vi "Mouse Breathing Monitor V6.vi"() -> ()   [LabVIEW 2017]
uses:
  <vilib>/Utility/error.llb/DialogType.ctl
  <vilib>/Utility/sysdir.llb/System Directory Type.ctl
  C:/Program Files (x86)/National Instruments/LabVIEW 2017/vi.lib/ULx/ULx_LV.dll
  Program Files (x86)/National Instruments/LabVIEW 2017/vi.lib/ULx/ULx_LV.dll
  <vilib>/Analysis/baseanly.llb/Mean (DBL).vi
  <vilib>/ULx/Create Channel.llb/ULx Create Channel (AI-Voltage-Basic).vi
  <vilib>/ULx/Timing.llb/ULx Timing (Sample Clock).vi
  <vilib>/ULx/Read.llb/ULx Read (Analog 2D DBL NChan NSamp).vi
  <vilib>/Analysis/NI_AALBase.lvlib
panel:
  in  "CH 2 Calibration Volume (mL)":dbl min=0.0 max=0.5 format="%#_13g"
  in  "CH 1 Calibration Volume (mL)":dbl min=0.0 max=0.5 format="%#_13g"
  in  "CH2 Cuff Alarm Threshold":dbl=3.0
  out "CH2 Cuff Alarm":bool
  in  "CH1 Cuff Alarm Threshold":dbl=3.0
  out "CH1 Cuff Alarm":bool
  out "CH1 Cuff":dbl format="%0.2f"
  out "CH2 Cuff":dbl format="%0.2f"
  in  "Invert Signal?":bool=TRUE
  in  "CH2 Log Button":bool
  in  "CH2 Logging":bool
  in  "CH2 Record\nButton":bool
  in  "CH1 Record\nButton":bool
  in  "CH2 Mouse ID":string
  in  "CH2 Recording":bool
  in  "CH1 Recording":bool
  in  "CH2 refnum":refnum<file>
  in  "Seconds to Display":i32=5 min=1
  in  "CH1 Logging":bool
  in  "CH1 Log Button":bool
  in  "CH1 refnum":refnum<file>
  in  "Exit":bool
  in  "CH1 Mouse ID":string
  in  "Stop":bool
  out "CH2 Chart":dbl[](graph)=[4.998778820037842, 4.998778820037842, 4.998778820037842, 5.00122082256712, 4.998778820037842, 4.998778820037842, 4.998778820037842, 4.998778820037842, 4.998778820037842, 5.00122082256712]
  out "CH1 Chart":dbl[](graph)=[4.998778820037842, 5.00122082256712, 4.998778820037842, 4.998778820037842, 5.00122082256712, 4.998778820037842, 5.00122082256712, 4.998778820037842, 4.998778820037842, 5.00122082256712]
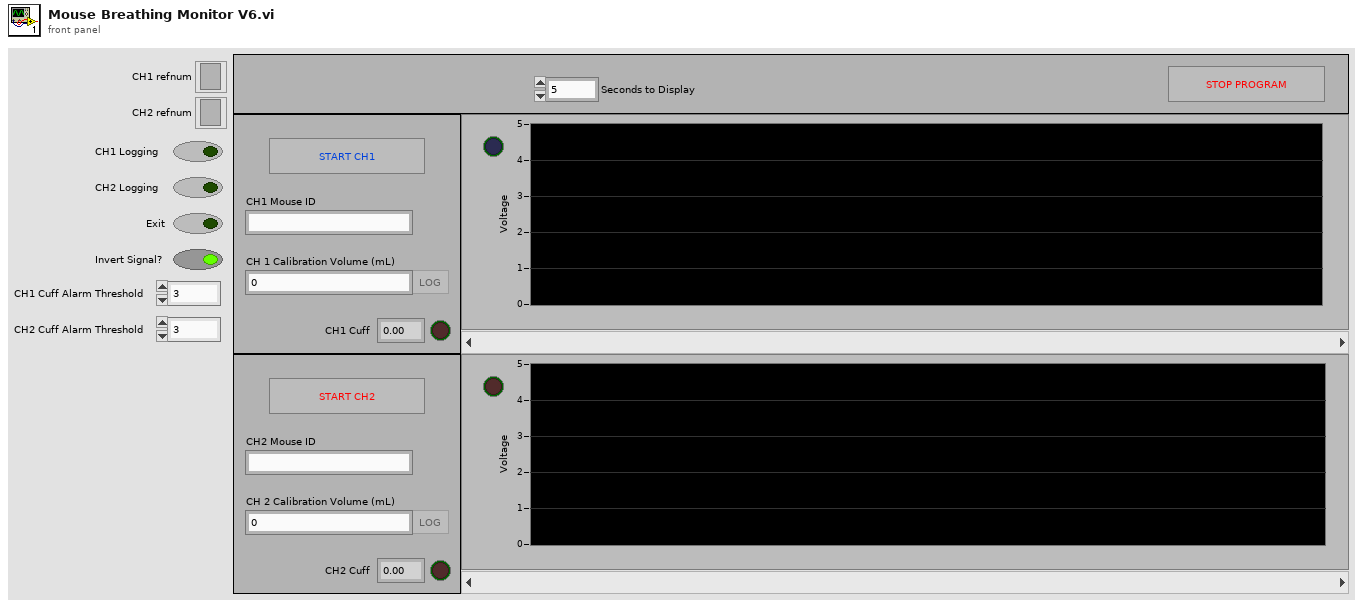
[diagram p1: front panel]
types:
  T1 = typedef "System Directory Type.ctl" = i32
  T2 = typedef "DialogType.ctl" = u16
  T3 = enum8{"Enabled", "Disabled", "Disabled and Grayed Out"}
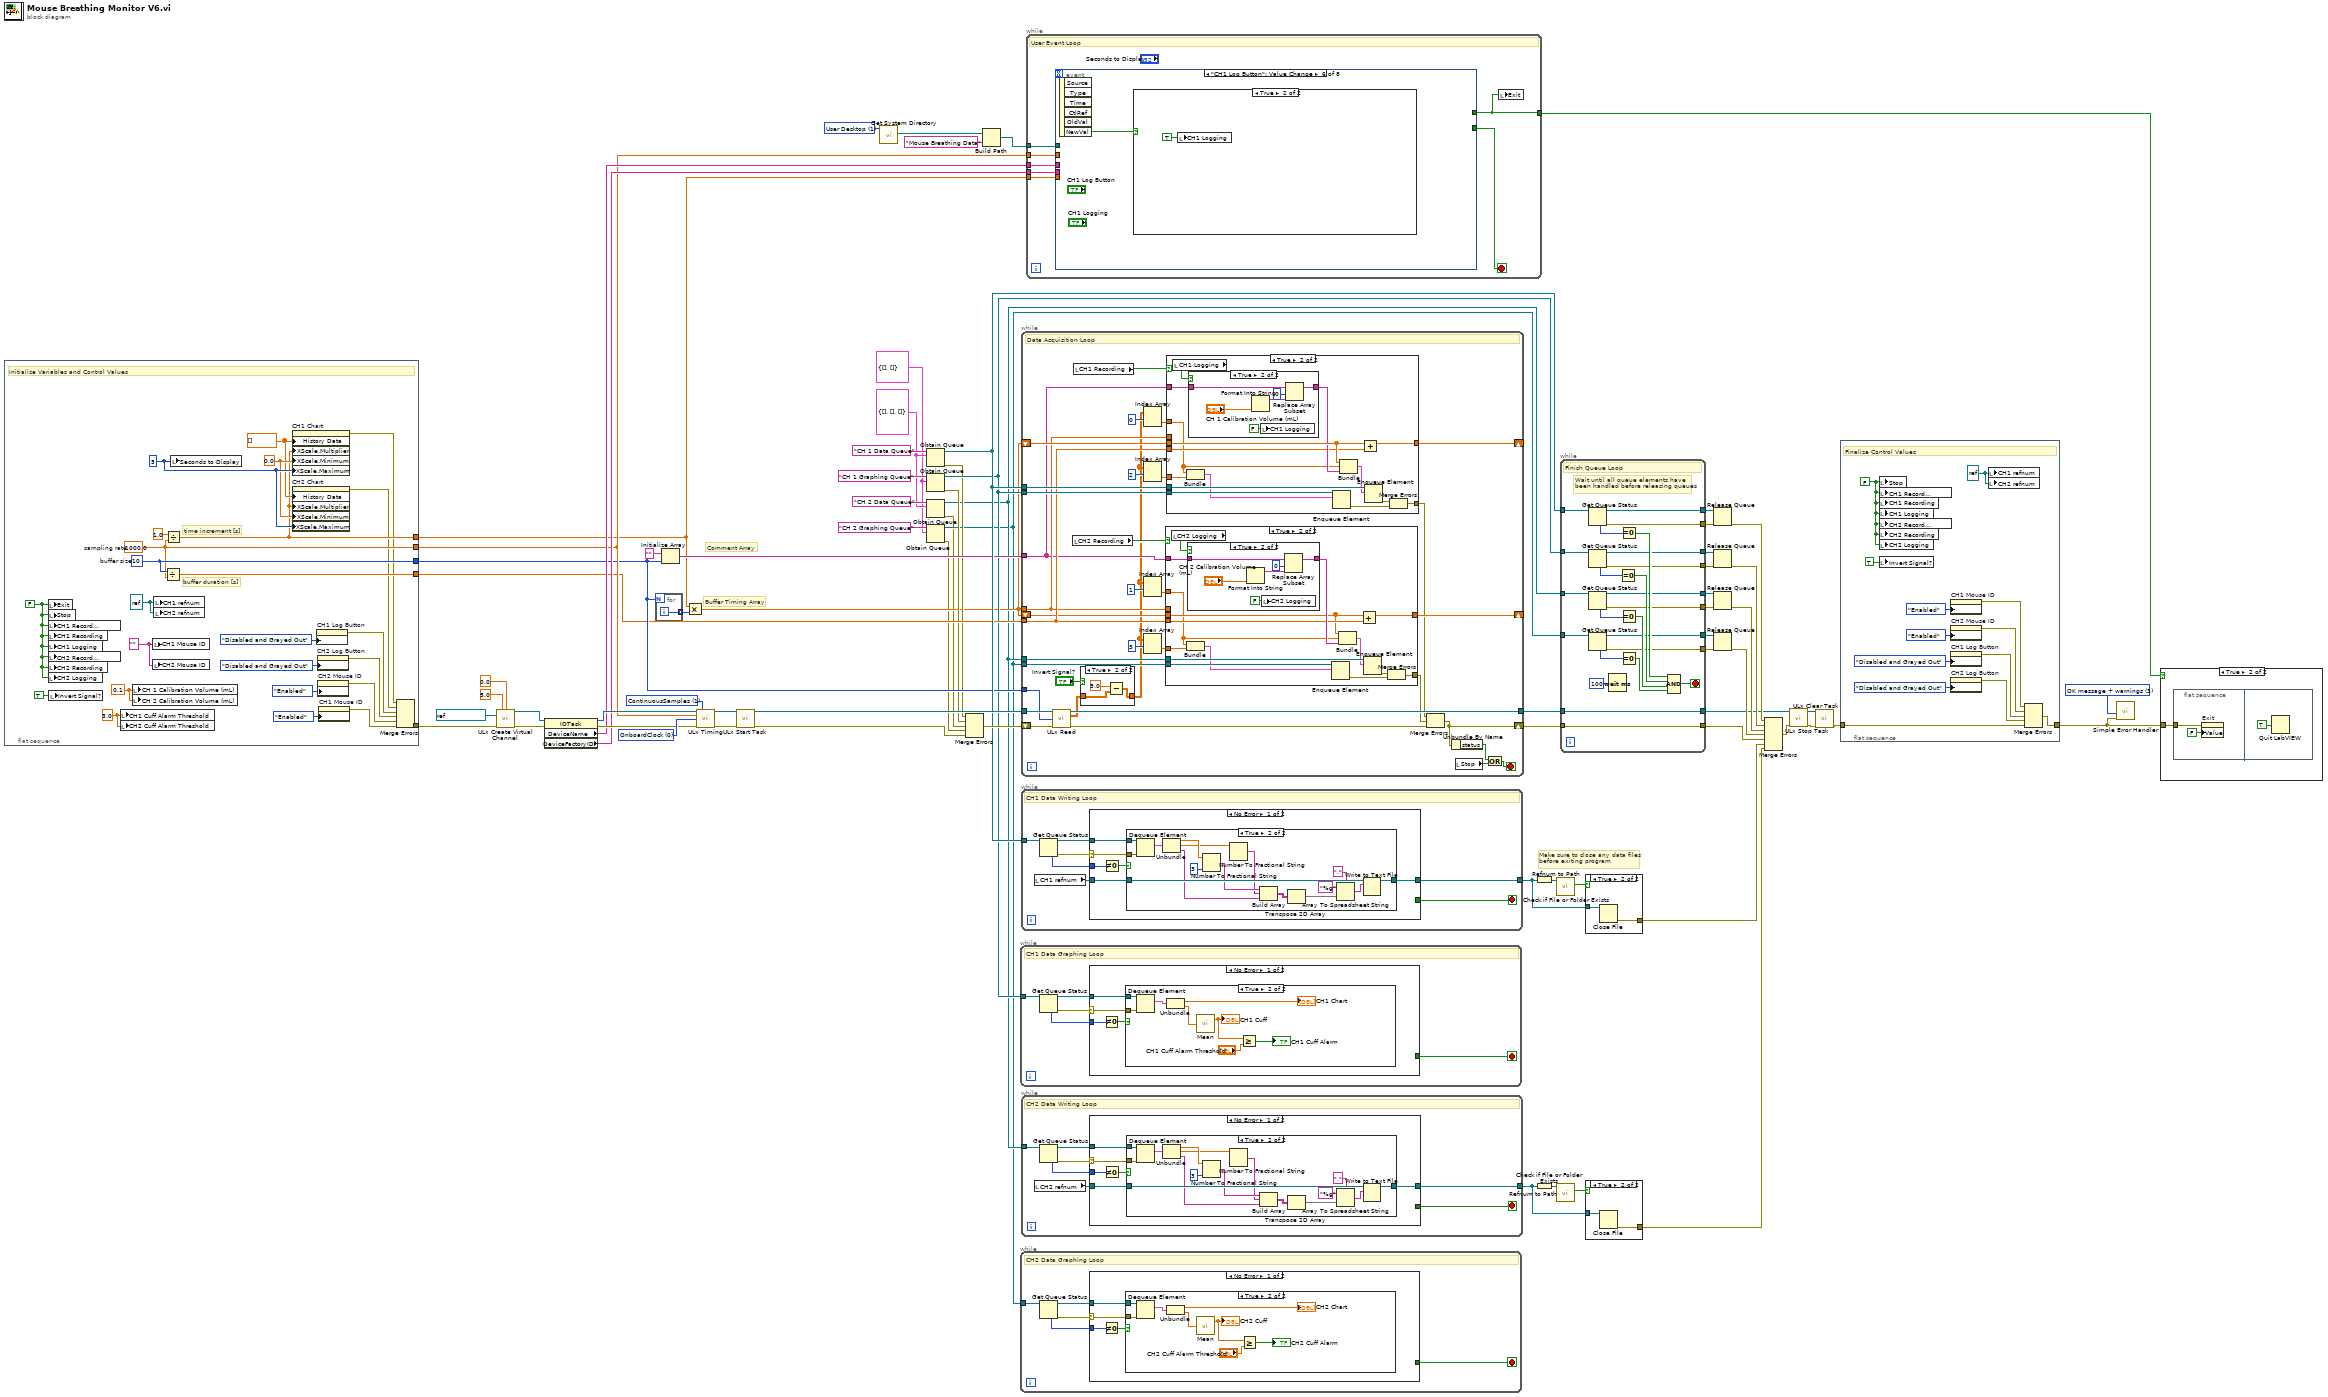
[diagram p0: block diagram]
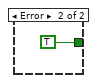
[diagram p4: hidden frame]
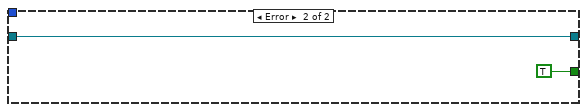
[diagram p6: hidden frame]
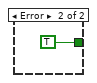
[diagram p8: hidden frame]
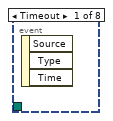
[diagram p11: hidden frame]
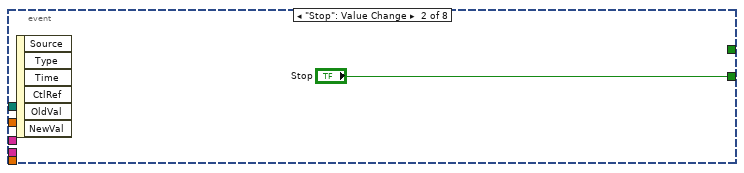
[diagram p12: hidden frame]
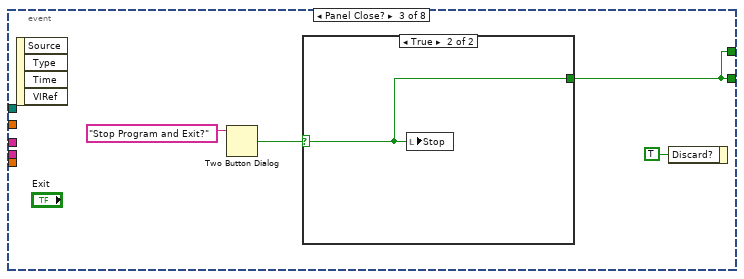
[diagram p13: hidden frame]
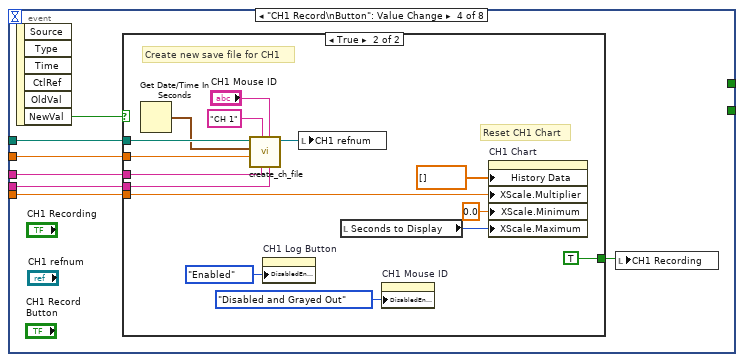
[diagram p15: hidden frame]
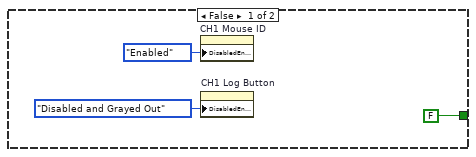
[diagram p16: hidden frame]
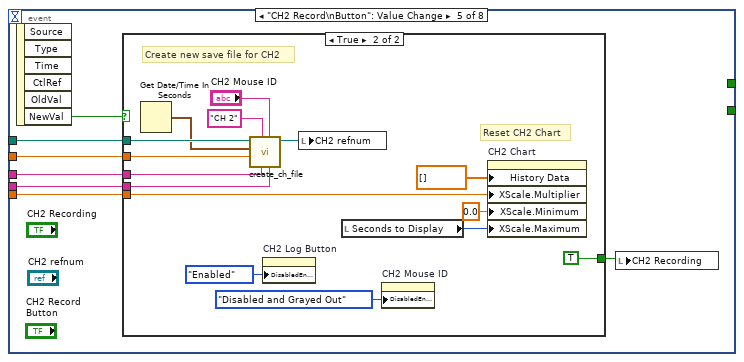
[diagram p17: hidden frame]
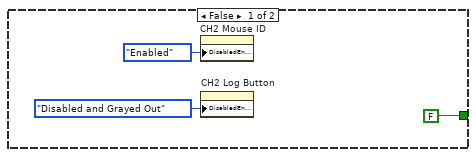
[diagram p18: hidden frame]
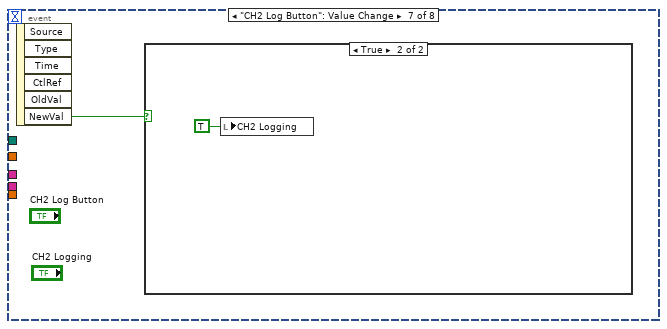
[diagram p20: hidden frame]
diagram:
  w1 = cluster{dbl[], dbl[]} {[], []}
  w32 = cluster{dbl[], dbl[], string[]} {[], [], []}
  w61 = T1 1 items=["User Home"=0, "User Desktop"=1, "User Documents"=2, "User Application Data"=3, "User Preferences"=4, "User Temporary"=5, "Public Documents"=6, "Public Application Data"=7, "Public Preferences"=8, "Public Cache"=13, "System Core Libraries"=9, "System Installed Libraries"=10, "Application Files"=11, "Boot Volume Root"=12] ("system directory type")
  w62 = 1 items=["FiniteSamples", "ContinuousSamples"] ("sample mode")
  w63 = 0 items=["OnboardClock", "ExternalClock", "NoClock"] ("clock source")
  w71 = T2 3 items=["no dialog", "OK message", "continue or stop message", "OK message + warnings", "continue/stop + warnings"] ("type of dialog (OK msg:1)")
  # "Make sure to close any data files\nbefore exiting program"
  # "Comment Array"
  # "Buffer Timing Array"
  n1 = flat-sequence {
    tunnel: [w89] -> w50
    tunnel: [w96] -> w45
    tunnel: [w97] -> w44
    tunnel: [w79] -> w43
    tunnel: [w95] -> w42
    frame #0 {
      w75 = 0.1 ("CH 1 Calibration Volume (mL)")
      w76 = 3.0
      w84 = refnum<file> refnum ("CH 1 refnum")
      w81 = 0.0 ("X Scale.Range:Minimum")
      w82 = 5 ("Seconds to Display")
      w80 = dbl[] [] ("CH1 Chart")
      w85 = "" ("CH 1 Mouse ID")
      w92 = FALSE ("Exit")
      w97 = 10  # buffer size
      w96 = 1000.0  # sampling rate
      # "buffer duration [s]"
      # "time increment [s]"
      # "Initialize Variables and Control Values"
      n2 = local write "Exit"(w92) -> ()
      n3 = local write "Stop"(w92) -> ()
      n4 = local write "CH1 Record\nButton"(w92) -> ()
      n5 = local write "CH1 Recording"(w92) -> ()
      n6 = local write "CH1 Logging"(w92) -> ()
      n7 = local write "CH2 Record\nButton"(w92) -> ()
      n8 = local write "CH2 Recording"(w92) -> ()
      n9 = local write "CH2 Logging"(w92) -> ()
      n10 = local write "Invert Signal?"(TRUE ("Invert Signal?")) -> ()
      n11 = local write "CH1 Cuff Alarm Threshold"(w76) -> ()
      n12 = local write "CH2 Cuff Alarm Threshold"(w76) -> ()
      n13 = local write "CH 1 Calibration Volume (mL)"(w75) -> ()
      n14 = local write "CH 2 Calibration Volume (mL)"(w75) -> ()
      n15 = local write "CH1 Mouse ID"(w85) -> ()
      n16 = local write "CH2 Mouse ID"(w85) -> ()
      n17 = local write "CH1 refnum"(w84) -> ()
      n18 = local write "CH2 refnum"(w84) -> ()
      n19 = Divide(x=w97, y=w96) -> (x/y=w95:dbl)
      n20 = Divide(x=1.0, y=w96) -> (x/y=w79:dbl)
      n21 = local write "Seconds to Display"(w82) -> ()
      n22 = property on="CH1 Chart" class="WFChart (strict)"("History Data"=w80, "XScale.Multiplier"=w79, "XScale.Minimum"=w81, "XScale.Maximum"=w82) -> (error out=w78:errorcluster)  [unwired: 2 in, 1 out]
      n23 = property on="CH2 Chart" class="WFChart (strict)"("History Data"=w80, "XScale.Multiplier"=w79, "XScale.Minimum"=w81, "XScale.Maximum"=w82) -> (error out=w77:errorcluster)  [unwired: 2 in, 1 out]
      n24 = property on="CH1 Log Button" class="Bool"("DisabledEnum"=T3."Disabled and Grayed Out" ("Disabled")) -> (error out=w86:errorcluster)  [unwired: 2 in, 1 out]
      n25 = property on="CH2 Log Button" class="Bool"("DisabledEnum"=T3."Disabled and Grayed Out" ("Disabled")) -> (error out=w87:errorcluster)  [unwired: 2 in, 1 out]
      n26 = property on="CH2 Mouse ID" class="Str"("DisabledEnum"=T3."Enabled" ("Disabled")) -> (error out=w88:errorcluster)  [unwired: 2 in, 1 out]
      n27 = property on="CH1 Mouse ID" class="Str"("DisabledEnum"=T3."Enabled" ("Disabled")) -> (error out=w99:errorcluster)  [unwired: 2 in, 1 out]
      n28 = Merge Errors(w78, w77, w86, w87, w88, w99) -> (w89:errorcluster)
    }
  }
  n29 = call-poly <vilib>:"ULx Create Virtual Channel.vi"("maximum value"=5.0, "minimum value"=0.0, "physical channels"=refnum<k21> "Dev0/Ai0:3", "error in"=w50) -> ("task out"=w57:refnum<k24>, "error out"=w55:errorcluster)  [unwired: 10 in]
  n30 = property class="IOTask"(reference=w57, error in=w55) -> (reference out=w56:refnum<k24>, error out=w54:errorcluster, "DeviceName"=w53:string, "DeviceFactoryID"=w52:string)
  n31 = for {
    N: w44 -> [_]
    tunnel: [w100] -> w48 mode=indexing
    i -> [w100]
  }
  n32 = Initialize Array("", w44) -> (w46:string[])
  n33 = Multiply(x=w43, y=w48) -> (x*y=w20:dbl[])
  n34 = call-poly <vilib>:"ULx Timing.vi"("task in"=w56, "sample mode"=w62, "rate"=w45, "clock source"=w63, "error in"=w54) -> ("task out"=w65:refnum<k24>, "error out"=w64:errorcluster)  [unwired: 9 in]
  n35 = call <vilib>:"ULx Start Task.vi"("task in"=w65, "error in"=w64) -> ("task out"=w74:refnum<k24>, "error out"=w3:errorcluster)  [unwired: 12 in]
  n36 = call <vilib>:"Get System Directory.vi"("system directory type"=w61) -> ("system directory"=w59:path)  [unwired: 10 in]
  n37 = Obtain Queue(name (unnamed)="CH 1 Data Queue", element data type=w32) -> (queue out=w51:refnum<queue>, error out=w30:errorcluster)  [unwired: 3 in, 1 out]
  n38 = Obtain Queue(name (unnamed)="CH 1 Graphing Queue", element data type=w1) -> (queue out=w31:refnum<queue>, error out=w29:errorcluster)  [unwired: 3 in, 1 out]
  n39 = Obtain Queue(name (unnamed)="CH 2 Data Queue", element data type=w32) -> (queue out=w19:refnum<queue>, error out=w5:errorcluster)  [unwired: 3 in, 1 out]
  n40 = Obtain Queue(name (unnamed)="CH 2 Graphing Queue", element data type=w1) -> (queue out=w18:refnum<queue>, error out=w4:errorcluster)  [unwired: 3 in, 1 out]
  n41 = Merge Errors(w30, w29, w5, w4, w3) -> (w66:errorcluster)
  n42 = Build Path(base path=w59, name or relative path="Mouse Breathing Data") -> (appended path=w58:path)
  n43 = while {
    tunnel: w31 -> [w101]
    stop <- w103 stop-if-true
    # "CH1 Data Graphing Loop"
    n44 = Get Queue Status(queue=w101) -> (queue out=w105:refnum<queue>, error out=w104:errorcluster, # elements in queue=w102:i32)  [unwired: 2 in, 5 out]
    n45 = case shown="No Error" w104 {
      selector: w104 -> [w108 _]
      tunnel: w105 -> [w109 _]
      tunnel: [_ TRUE] -> w103
      tunnel: w102 -> [w107 _]
      frame No Error {
        n46 = Not Equal To 0?(x=w107) -> (x != 0?=w106:bool)
        n47 = case shown="True" w106 {
          tunnel: w109 -> [_ w117]
          tunnel: w108 -> [_ w116]
          frame False {
            # "No data in queue. Do nothing."
          }
          frame True {
            n48 = Dequeue Element(queue=w117, error in (no error)=w116) -> (element=w115:cluster{dbl[], dbl[]})  [unwired: 1 in, 3 out]
            n49 = Unbundle(w115) -> (→"CH1 Chart":dbl[], w113:dbl[])
            n50 = call-poly <vilib>:"Mean.vi"("X"=w113) -> ("mean"=w112:dbl)  [unwired: 1 out]
            "CH1 Cuff" <- w112
            n51 = Greater Or Equal?(x=w112, y="CH1 Cuff Alarm Threshold") -> (x >= y?=→"CH1 Cuff Alarm":bool)
          }
        }
      }
      frame Error {
      }
    }
  }
  n52 = while {
    tunnel: w18 -> [w119]
    stop <- w121 stop-if-true
    # "CH2 Data Graphing Loop"
    n53 = Get Queue Status(queue=w119) -> (queue out=w123:refnum<queue>, error out=w122:errorcluster, # elements in queue=w120:i32)  [unwired: 2 in, 5 out]
    n54 = case shown="No Error" w122 {
      selector: w122 -> [w126 _]
      tunnel: w123 -> [w127 _]
      tunnel: [_ TRUE] -> w121
      tunnel: w120 -> [w125 _]
      frame No Error {
        n55 = Not Equal To 0?(x=w125) -> (x != 0?=w124:bool)
        n56 = case shown="True" w124 {
          tunnel: w127 -> [_ w135]
          tunnel: w126 -> [_ w134]
          frame False {
            # "No data in queue. Do nothing."
          }
          frame True {
            n57 = Dequeue Element(queue=w135, error in (no error)=w134) -> (element=w133:cluster{dbl[], dbl[]})  [unwired: 1 in, 3 out]
            n58 = Unbundle(w133) -> (→"CH2 Chart":dbl[], w131:dbl[])
            n59 = call-poly <vilib>:"Mean.vi"("X"=w131) -> ("mean"=w130:dbl)  [unwired: 1 out]
            "CH2 Cuff" <- w130
            n60 = Greater Or Equal?(x=w130, y="CH2 Cuff Alarm Threshold") -> (x >= y?=→"CH2 Cuff Alarm":bool)
          }
        }
      }
      frame Error {
      }
    }
  }
  n61 = while {
    tunnel: w51 -> [w142]
    tunnel: [w143] -> w38
    stop <- w138 stop-if-true
    # "CH1 Data Writing Loop"
    n62 = local read "CH1 refnum"() -> (w139:refnum<file>)
    n63 = Get Queue Status(queue=w142) -> (queue out=w141:refnum<queue>, error out=w140:errorcluster, # elements in queue=w137:i32)  [unwired: 2 in, 5 out]
    n64 = case shown="No Error" w140 {
      selector: w140 -> [w147 _]
      tunnel: [w149 w168] -> w143
      tunnel: w141 -> [w148 _]
      tunnel: w139 -> [w146 w168]
      tunnel: [_ TRUE] -> w138
      tunnel: w137 -> [w145 _]
      frame No Error {
        n65 = Not Equal To 0?(x=w145) -> (x != 0?=w144:bool)
        n66 = case shown="True" w144 {
          tunnel: [w150 w166] -> w149
          tunnel: w148 -> [_ w165]
          tunnel: w147 -> [_ w164]
          tunnel: w146 -> [w150 w163]
          frame False {
            # "No data in queue. Do nothing."
          }
          frame True {
            n67 = Dequeue Element(queue=w165, error in (no error)=w164) -> (element=w159:cluster{dbl[], dbl[], string[]})  [unwired: 1 in, 3 out]
            n68 = Unbundle(w159) -> (w158:dbl[], w157:dbl[], w153:string[])
            n69 = Number To Fractional String(number=w158, precision (6)=i16 3) -> (F-format string=w155:string[])  [unwired: 2 in]
            n70 = Number To Fractional String(number=w157) -> (F-format string=w154:string[])  [unwired: 3 in]
            n71 = Build Array(w155, w154, w153) -> (w152:string[][])
            n72 = Transpose 2D Array(2D array=w152) -> (transposed array=w151:string[][])
            n73 = Array To Spreadsheet String(delimiter (Tab)=",", array=w151, 3:"%g" ("format string")) -> (spreadsheet string=w162:string)
            n74 = Write to Text File(file (use dialog)=w163, text=w162) -> (refnum out=w166:refnum<file>)  [unwired: 2 in, 2 out]
          }
        }
      }
      frame Error {
      }
    }
  }
  n75 = while {
    tunnel: w19 -> [w174]
    tunnel: [w175] -> w15
    stop <- w170 stop-if-true
    # "CH2 Data Writing Loop"
    n76 = local read "CH2 refnum"() -> (w171:refnum<file>)
    n77 = Get Queue Status(queue=w174) -> (queue out=w173:refnum<queue>, error out=w172:errorcluster, # elements in queue=w169:i32)  [unwired: 2 in, 5 out]
    n78 = case shown="No Error" w172 {
      selector: w172 -> [w179 _]
      tunnel: [w181 w200] -> w175
      tunnel: w173 -> [w180 _]
      tunnel: w171 -> [w178 w200]
      tunnel: [_ TRUE] -> w170
      tunnel: w169 -> [w177 _]
      frame No Error {
        n79 = Not Equal To 0?(x=w177) -> (x != 0?=w176:bool)
        n80 = case shown="True" w176 {
          tunnel: [w182 w198] -> w181
          tunnel: w180 -> [_ w197]
          tunnel: w179 -> [_ w196]
          tunnel: w178 -> [w182 w195]
          frame False {
            # "No data in queue. Do nothing."
          }
          frame True {
            n81 = Dequeue Element(queue=w197, error in (no error)=w196) -> (element=w191:cluster{dbl[], dbl[], string[]})  [unwired: 1 in, 3 out]
            n82 = Unbundle(w191) -> (w190:dbl[], w189:dbl[], w185:string[])
            n83 = Number To Fractional String(number=w190, precision (6)=i16 3) -> (F-format string=w187:string[])  [unwired: 2 in]
            n84 = Number To Fractional String(number=w189) -> (F-format string=w186:string[])  [unwired: 3 in]
            n85 = Build Array(w187, w186, w185) -> (w184:string[][])
            n86 = Transpose 2D Array(2D array=w184) -> (transposed array=w183:string[][])
            n87 = Array To Spreadsheet String(delimiter (Tab)=",", array=w183, 3:"%g" ("format string")) -> (spreadsheet string=w194:string)
            n88 = Write to Text File(file (use dialog)=w195, text=w194) -> (refnum out=w198:refnum<file>)  [unwired: 2 in, 2 out]
          }
        }
      }
      frame Error {
      }
    }
  }
  n89 = while {
    tunnel: [w235] -> w9
    tunnel: w74 -> [w234]
    tunnel: w51 -> [w232]
    shift-right: [w220] -> w7
    shift-left: w66 -> [w233]
    tunnel: w20 -> [w216]
    tunnel: w44 -> [w224]
    shift-right: [w222] -> _
    shift-left: w20 -> [w223]
    tunnel: w42 -> [w217]
    tunnel: w46 -> [w210]
    tunnel: w31 -> [w221]
    shift-right: [w214] -> _
    shift-left: w20 -> [w215]
    tunnel: w19 -> [w212]
    tunnel: w18 -> [w211]
    stop <- w231 stop-if-true
    # "Data Acquisition Loop"
    n90 = call-poly <vilib>:"ULx Read.vi"("task in"=w234, "number of samples per channel"=w224, "error in"=w233) -> ("task out"=w235:refnum<k24>, "data"=w206:dbl[][], "error out"=w219:errorcluster)  [unwired: 10 in]
    n91 = local read "CH2 Recording"() -> (w218:bool)
    n92 = local read "CH1 Recording"() -> (w225:bool)
    n93 = case shown="True" "Invert Signal?" {
      tunnel: w206 -> [w236 w238]
      tunnel: [w236 w239] -> w201
      frame False {
      }
      frame True {
        n94 = Subtract(x=5.0, y=w238) -> (x-y=w239:dbl[][])
      }
    }
    n95 = Index Array(array=w201, index (row)=0) -> (element=w202:dbl[])  [unwired: 1 in]
    n96 = Index Array(array=w201, index (row)=2) -> (element=w226:dbl[])  [unwired: 1 in]
    n97 = Index Array(array=w201, index (row)=1) -> (element=w203:dbl[])  [unwired: 1 in]
    n98 = Index Array(array=w201, index (row)=3) -> (element=w213:dbl[])  [unwired: 1 in]
    n99 = case shown="True" w218 {
      tunnel: [_ w251] -> w208
      tunnel: [w240 w254] -> w214
      tunnel: w217 -> [_ w249]
      tunnel: w216 -> [w240 _]
      tunnel: w215 -> [_ w246]
      tunnel: w213 -> [_ w241]
      tunnel: w212 -> [_ w248]
      tunnel: w211 -> [_ w247]
      tunnel: w210 -> [_ w244]
      tunnel: w203 -> [_ w242]
      frame False {
      }
      frame True {
        n100 = local read "CH2 Logging"() -> (w252:bool)
        n101 = Bundle("data"=w242, "data"=w241) -> (w243:cluster{"data":dbl[], "data":dbl[]})  [unwired: 1 in]
        n102 = case shown="True" w252 {
          tunnel: [w256 w262] -> w253
          tunnel: w244 -> [w256 w259]
          frame False {
          }
          frame True {
            n103 = Format Into String("CH 2 Calibration Volume (mL)") -> (resulting string=w258:string)  [unwired: 3 in, 1 out]
            n104 = local write "CH2 Logging"(FALSE ("CH1 Log")) -> ()
            n105 = Replace Array Subset(array=w259, new element=w258, index=0) -> (w262:string[])
          }
        }
        n106 = Enqueue Element(queue=w247, element=w243) -> (error out=w250:errorcluster)  [unwired: 2 in, 2 out]
        n107 = Bundle(w246, "data"=w242, w253) -> (w245:cluster{dbl[], "data":dbl[], string[]})  [unwired: 1 in]
        n108 = Add(x=w246, y=w249) -> (x+y=w254:dbl[])
        n109 = Enqueue Element(queue=w248, element=w245) -> (error out=w255:errorcluster)  [unwired: 2 in, 2 out]
        n110 = Merge Errors(w255, w250) -> (w251:errorcluster)
      }
    }
    n111 = case shown="True" w225 {
      tunnel: w232 -> [_ w278]
      tunnel: w226 -> [_ w265]
      tunnel: [_ w268] -> w209
      tunnel: w223 -> [_ w275]
      tunnel: [w263 w276] -> w222
      tunnel: w216 -> [w263 _]
      tunnel: w217 -> [_ w272]
      tunnel: w210 -> [_ w271]
      tunnel: w221 -> [_ w269]
      tunnel: w202 -> [_ w266]
      frame False {
      }
      frame True {
        n112 = local read "CH1 Logging"() -> (w270:bool)
        n113 = Bundle("data"=w266, "data"=w265) -> (w264:cluster{"data":dbl[], "data":dbl[]})  [unwired: 1 in]
        n114 = case shown="True" w270 {
          tunnel: [w279 w284] -> w274
          tunnel: w271 -> [w279 w285]
          frame False {
          }
          frame True {
            n115 = Format Into String("CH 1 Calibration Volume (mL)") -> (resulting string=w280:string)  [unwired: 3 in, 1 out]
            n116 = local write "CH1 Logging"(FALSE ("CH1 Log")) -> ()
            n117 = Replace Array Subset(array=w285, new element=w280, index=0) -> (w284:string[])
          }
        }
        n118 = Enqueue Element(queue=w269, element=w264) -> (error out=w267:errorcluster)  [unwired: 2 in, 2 out]
        n119 = Bundle(w275, "data"=w266, w274) -> (w273:cluster{dbl[], "data":dbl[], string[]})  [unwired: 1 in]
        n120 = Add(x=w275, y=w272) -> (x+y=w276:dbl[])
        n121 = Enqueue Element(queue=w278, element=w273) -> (error out=w277:errorcluster)  [unwired: 2 in, 2 out]
        n122 = Merge Errors(w277, w267) -> (w268:errorcluster)
      }
    }
    n123 = Merge Errors(w209, w208, w219) -> (w220:errorcluster)
    n124 = Unbundle By Name(w220) -> ("status"=w230:bool)
    n125 = local read "Stop"() -> (w229:bool)
    n126 = Or(x=w230, y=w229) -> (x .or. y?=w231:bool)
  }
  n127 = while {
    tunnel: w58 -> [w291]
    tunnel: w53 -> [w290]
    tunnel: w52 -> [w289]
    tunnel: w45 -> [w288]
    tunnel: w43 -> [w287]
    tunnel: [w286] -> w2
    stop <- w292 stop-if-true
    # "User Event Loop"
    n128 = event shown="[5] \"CH1 Log Button\": Value Change" {
      selector: _ -> [_ _ _ _ _ _ _ _]
      dyn-events: _ -> [_ _ _ _ _ _ _ _]
      timeout: _ -> [_ _ _ _ _ _ _ _]
      tunnel: [_ "Stop" w294 _ _ _ _ _] -> w292
      tunnel: w291 -> [_ _ _ w305 w330 _ _ _]
      tunnel: w290 -> [_ _ _ w304 w329 _ _ _]
      tunnel: w289 -> [_ _ _ w303 w328 _ _ _]
      tunnel: w288 -> [_ _ _ w302 w327 _ _ _]
      tunnel: w287 -> [_ _ _ w300 w325 _ _ _]
      tunnel: [_ _ w294 _ _ _ _ _] -> w286
      event Timeout {
        n129 = event-data() -> ()  [unwired: 1 in, 3 out]
      }
      event "Stop": Value Change {
        n130 = event-data() -> ()  [unwired: 1 in, 6 out]
      }
      event Panel Close? {
        n131 = event-data() -> ()  [unwired: 1 in, 4 out]
        n132 = Two Button Dialog(message="Stop Program and Exit?") -> (T button?=w295:bool)  [unwired: 2 in]
        n133 = case shown="True" w295 {
          selector: w295 -> [w298 w299]
          tunnel: [w298 w299] -> w294
          frame False {
          }
          frame True {
            n134 = local write "Stop"(w299) -> ()
          }
        }
        n135 = event-data("Discard?"=TRUE) -> ()  [unwired: 1 in, 1 out]
      }
      event "CH1 Record\nButton": Value Change {
        n136 = event-data() -> ("NewVal"=w306:bool)  [unwired: 1 in, 5 out]
        n137 = case shown="True" w306 {
          tunnel: w305 -> [_ w320]
          tunnel: w304 -> [_ w317]
          tunnel: w303 -> [_ w316]
          tunnel: w302 -> [_ w318]
          tunnel: [FALSE ("CH1 Logging") TRUE ("CH1 Logging")] -> w301
          tunnel: w300 -> [_ w313]
          frame False {
            n138 = property on="CH1 Mouse ID" class="Str"("DisabledEnum"=T3."Enabled" ("Disabled")) -> ()  [unwired: 2 in, 2 out]
            n139 = property on="CH1 Log Button" class="Bool"("DisabledEnum"=T3."Disabled and Grayed Out" ("Disabled")) -> ()  [unwired: 2 in, 2 out]
          }
          frame True {
            # "Reset CH1 Chart"
            # "Create new save file for CH1"
            n140 = Get Date/Time In Seconds() -> (seconds since 1Jan1904=w319:timestamp)
            n141 = call "create_ch_file.vi"("device factory id"=w316, "mouse id"="CH1 Mouse ID", "device name"=w317, "channel name"="CH 1", "sampling rate"=w318, "time stamp"=w319, "appended path"=w320) -> ("refnum out"=w315:refnum<file>)  [unwired: 3 in, 1 out]
            n142 = property on="CH1 Log Button" class="Bool"("DisabledEnum"=T3."Enabled" ("Disabled")) -> ()  [unwired: 2 in, 2 out]
            n143 = local write "CH1 refnum"(w315) -> ()
            n144 = local read "Seconds to Display"() -> (w310:i32)
            n145 = property on="CH1 Mouse ID" class="Str"("DisabledEnum"=T3."Disabled and Grayed Out" ("Disabled")) -> ()  [unwired: 2 in, 2 out]
            n146 = property on="CH1 Chart" class="WFChart (strict)"("History Data"=dbl[] [] ("CH1 Chart"), "XScale.Multiplier"=w313, "XScale.Minimum"=0.0 ("X Scale.Range:Minimum"), "XScale.Maximum"=w310) -> ()  [unwired: 2 in, 2 out]
          }
        }
        n147 = local write "CH1 Recording"(w301) -> ()
      }
      event "CH2 Record\nButton": Value Change {
        n148 = event-data() -> ("NewVal"=w331:bool)  [unwired: 1 in, 5 out]
        n149 = case shown="True" w331 {
          tunnel: w330 -> [_ w345]
          tunnel: w329 -> [_ w342]
          tunnel: w328 -> [_ w341]
          tunnel: w327 -> [_ w343]
          tunnel: [FALSE ("CH1 Logging") TRUE ("CH1 Logging")] -> w326
          tunnel: w325 -> [_ w338]
          frame False {
            n150 = property on="CH2 Mouse ID" class="Str"("DisabledEnum"=T3."Enabled" ("Disabled")) -> ()  [unwired: 2 in, 2 out]
            n151 = property on="CH2 Log Button" class="Bool"("DisabledEnum"=T3."Disabled and Grayed Out" ("Disabled")) -> ()  [unwired: 2 in, 2 out]
          }
          frame True {
            # "Reset CH2 Chart"
            # "Create new save file for CH2"
            n152 = Get Date/Time In Seconds() -> (seconds since 1Jan1904=w344:timestamp)
            n153 = call "create_ch_file.vi"("device factory id"=w341, "mouse id"="CH2 Mouse ID", "device name"=w342, "channel name"="CH 2", "sampling rate"=w343, "time stamp"=w344, "appended path"=w345) -> ("refnum out"=w340:refnum<file>)  [unwired: 3 in, 1 out]
            n154 = property on="CH2 Log Button" class="Bool"("DisabledEnum"=T3."Enabled" ("Disabled")) -> ()  [unwired: 2 in, 2 out]
            n155 = local write "CH2 refnum"(w340) -> ()
            n156 = local read "Seconds to Display"() -> (w335:i32)
            n157 = property on="CH2 Mouse ID" class="Str"("DisabledEnum"=T3."Disabled and Grayed Out" ("Disabled")) -> ()  [unwired: 2 in, 2 out]
            n158 = property on="CH2 Chart" class="WFChart (strict)"("History Data"=dbl[] [] ("CH1 Chart"), "XScale.Multiplier"=w338, "XScale.Minimum"=0.0 ("X Scale.Range:Minimum"), "XScale.Maximum"=w335) -> ()  [unwired: 2 in, 2 out]
          }
        }
        n159 = local write "CH2 Recording"(w326) -> ()
      }
      event "CH1 Log Button": Value Change {
        n160 = event-data() -> ("NewVal"=w350:bool)  [unwired: 1 in, 5 out]
        n161 = case shown="True" w350 {
          frame False {
          }
          frame True {
            n162 = local write "CH1 Logging"(TRUE ("CH1 Log")) -> ()
          }
        }
      }
      event "CH2 Log Button": Value Change {
        n163 = event-data() -> ("NewVal"=w352:bool)  [unwired: 1 in, 5 out]
        n164 = case shown="True" w352 {
          frame False {
          }
          frame True {
            n165 = local write "CH2 Logging"(TRUE ("CH1 Log")) -> ()
          }
        }
      }
      event "Seconds to Display": Value Change {
        n166 = event-data() -> ("NewVal"=w362:i32, "OldVal"=w361:i32)  [unwired: 1 in]
        n167 = Subtract(x=w362, y=w361) -> (x-y=w356:i32)
        n168 = property on="CH1 Chart" class="WFChart (strict)"() -> (error out=w360:errorcluster, "XScale.Maximum"=w359:dbl)  [unwired: 2 in, 1 out]
        n169 = property on="CH2 Chart" class="WFChart (strict)"() -> (error out=w355:errorcluster, "XScale.Maximum"=w354:dbl)  [unwired: 2 in, 1 out]
        n170 = Add(x=w356, y=w359) -> (x+y=w358:dbl)
        n171 = Add(x=w356, y=w354) -> (x+y=w357:dbl)
        n172 = property on="CH1 Chart" class="WFChart (strict)"(error in=w360, "XScale.Maximum"=w358) -> ()  [unwired: 1 in, 2 out]
        n173 = property on="CH2 Chart" class="WFChart (strict)"(error in=w355, "XScale.Maximum"=w357) -> ()  [unwired: 1 in, 2 out]
      }
    }
    n174 = local write "Exit"(w286) -> ()
  }
  n175 = Refnum to Path(1:w38) -> (0:w40:path)
  n176 = Refnum to Path(1:w15) -> (0:w17:path)
  n177 = call <vilib>:"Check if File or Folder Exists.vi"("path"=w40) -> ("file or folder exists?"=w39:bool)  [unwired: 8 in, 2 out]
  n178 = call <vilib>:"Check if File or Folder Exists.vi"("path"=w17) -> ("file or folder exists?"=w16:bool)  [unwired: 8 in, 2 out]
  n179 = while {
    tunnel: w51 -> [w384]
    tunnel: w31 -> [w385]
    tunnel: w19 -> [w374]
    tunnel: w18 -> [w373]
    tunnel: [w372] -> w28
    tunnel: [w371] -> w27
    tunnel: [w370] -> w26
    tunnel: [w369] -> w25
    tunnel: [w368] -> w13
    tunnel: [w367] -> w12
    tunnel: [w366] -> w11
    tunnel: [w365] -> w10
    tunnel: w9 -> [w364]
    tunnel: [w364] -> w8
    tunnel: w7 -> [w363]
    tunnel: [w363] -> w6
    stop <- w381 stop-if-true
    # "Wait until all queue elements have\nbeen handled before releasing queues"
    # "Finish Queue Loop"
    n180 = Get Queue Status(queue=w384) -> (queue out=w372:refnum<queue>, error out=w368:errorcluster, # elements in queue=w383:i32)  [unwired: 2 in, 5 out]
    n181 = Get Queue Status(queue=w385) -> (queue out=w371:refnum<queue>, error out=w367:errorcluster, # elements in queue=w382:i32)  [unwired: 2 in, 5 out]
    n182 = Get Queue Status(queue=w374) -> (queue out=w370:refnum<queue>, error out=w366:errorcluster, # elements in queue=w378:i32)  [unwired: 2 in, 5 out]
    n183 = Get Queue Status(queue=w373) -> (queue out=w369:refnum<queue>, error out=w365:errorcluster, # elements in queue=w377:i32)  [unwired: 2 in, 5 out]
    n184 = Wait (ms)(milliseconds to wait=u32 100) -> ()  [unwired: 1 out]
    n185 = Equal To 0?(x=w382) -> (x = 0?=w379:bool)
    n186 = Equal To 0?(x=w383) -> (x = 0?=w380:bool)
    n187 = Equal To 0?(x=w378) -> (x = 0?=w376:bool)
    n188 = Equal To 0?(x=w377) -> (x = 0?=w375:bool)
    n189 = Compound Arithmetic op=AND(w380, w379, w376, w375) -> (w381:bool)
  }
  n190 = case shown="True" w39 {
    tunnel: w38 -> [_ w388]
    tunnel: [_ w387] -> w36
    frame False {
    }
    frame True {
      n191 = Close File(refnum=w388) -> (error out=w387:errorcluster)  [unwired: 1 in, 1 out]
    }
  }
  n192 = case shown="True" w16 {
    tunnel: w15 -> [_ w390]
    tunnel: [_ w389] -> w14
    frame False {
    }
    frame True {
      n193 = Close File(refnum=w390) -> (error out=w389:errorcluster)  [unwired: 1 in, 1 out]
    }
  }
  n194 = Release Queue(queue=w28, error in (no error)=w13) -> (error out=w24:errorcluster)  [unwired: 1 in, 2 out]
  n195 = Release Queue(queue=w27, error in (no error)=w12) -> (error out=w23:errorcluster)  [unwired: 1 in, 2 out]
  n196 = Release Queue(queue=w26, error in (no error)=w11) -> (error out=w22:errorcluster)  [unwired: 1 in, 2 out]
  n197 = Release Queue(queue=w25, error in (no error)=w10) -> (error out=w21:errorcluster)  [unwired: 1 in, 2 out]
  n198 = Merge Errors(w24, w23, w22, w21, w6, w36, w14) -> (w37:errorcluster)
  n199 = call <vilib>:"ULx Stop Task.vi"("error in"=w37, "task in"=w8) -> ("error out"=w73:errorcluster, "task out"=w72:refnum<k24>)  [unwired: 8 in]
  n200 = call <vilib>:"ULx Clear Task.vi"("task in"=w72, "error in"=w73) -> ("error out"=w49:errorcluster)  [unwired: 13 in]
  n201 = flat-sequence {
    tunnel: [w400] -> w41
    tunnel: w49 -> [w399]
    frame #0 {
      w398 = refnum<file> refnum ("CH 1 refnum")
      w402 = FALSE ("Exit")
      # "Finalize Control Values"
      n202 = local write "Stop"(w402) -> ()
      n203 = local write "CH1 Record\nButton"(w402) -> ()
      n204 = local write "CH1 Recording"(w402) -> ()
      n205 = local write "CH1 Logging"(w402) -> ()
      n206 = local write "CH2 Record\nButton"(w402) -> ()
      n207 = local write "CH2 Recording"(w402) -> ()
      n208 = local write "CH2 Logging"(w402) -> ()
      n209 = local write "Invert Signal?"(TRUE ("Invert Signal?")) -> ()
      n210 = property on="CH1 Mouse ID" class="Str"("DisabledEnum"=T3."Enabled" ("Disabled")) -> (error out=w395:errorcluster)  [unwired: 2 in, 1 out]
      n211 = property on="CH2 Mouse ID" class="Str"("DisabledEnum"=T3."Enabled" ("Disabled")) -> (error out=w394:errorcluster)  [unwired: 2 in, 1 out]
      n212 = property on="CH1 Log Button" class="Bool"("DisabledEnum"=T3."Disabled and Grayed Out" ("Disabled")) -> (error out=w393:errorcluster)  [unwired: 2 in, 1 out]
      n213 = property on="CH2 Log Button" class="Bool"("DisabledEnum"=T3."Disabled and Grayed Out" ("Disabled")) -> (error out=w392:errorcluster)  [unwired: 2 in, 1 out]
      n214 = local write "CH1 refnum"(w398) -> ()
      n215 = local write "CH2 refnum"(w398) -> ()
      n216 = Merge Errors(w395, w394, w393, w392, w399) -> (w400:errorcluster)
    }
  }
  n217 = call <vilib>:"Simple Error Handler.vi"("type of dialog (OK msg:1)"=w71, "error in (no error)"=w41) -> ()  [unwired: 3 in, 5 out]
  n218 = case shown="True" w2 {
    tunnel: w41 -> [_ w404]
    frame False {
    }
    frame True {
      n219 = flat-sequence {
        tunnel: w404 -> [w406]
        frame #0 {
          n220 = property on="Exit" class="Bool (strict)"(error in=w406, "Value"=FALSE ("Exit")) -> ()  [unwired: 1 in, 2 out]
        }
        frame #1 {
          n221 = Quit LabVIEW(quit? (T)=TRUE) -> ()
        }
      }
    }
  }
